vi "GetINIPathForAModule.vi"(8 "error in (no error)":errorcluster, 10 "Module":string, 11 "Test":refnum<class "Test.lvclass">) -> (0 "Error out":errorcluster, 2 "INI File":path, 3 "Test Class out":refnum<class "Test.lvclass">)   [LabVIEW 2018, in "Test.lvclass"]
uses:
  Test.lvclass
  Test.lvclass/Test.ctl
  Accessors/Read ErrorSeverity.vi
  Accessors/Read PluginPathArray.vi
  Accessors/Read PluginIndex.vi
  Accessors/Read ModuleList.vi
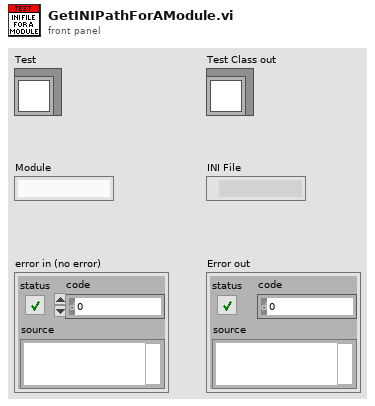
[diagram p1: front panel]
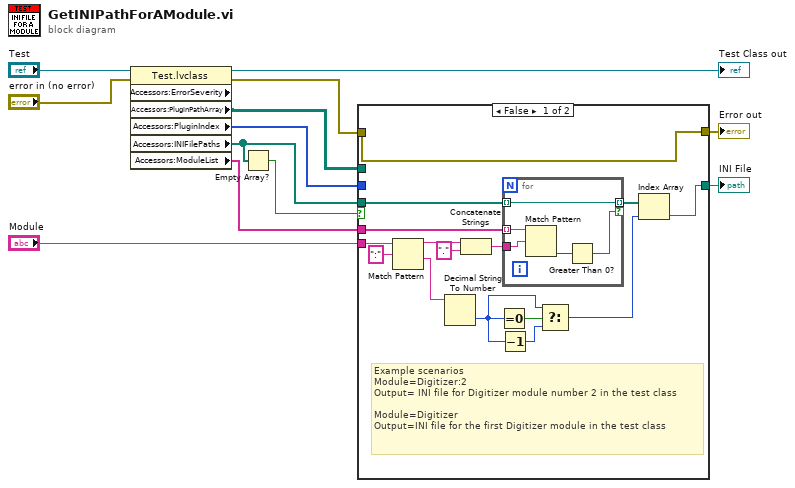
[diagram p0: block diagram]
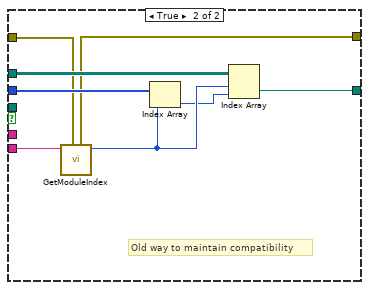
[diagram p2: hidden frame]
diagram:
  n1 = property class="Test.lvclass" props=["Accessors:ErrorSeverity", "Accessors:PluginPathArray", "Accessors:PluginIndex", "Accessors:INIFilePaths", "Accessors:ModuleList"](reference="Test", error in="error in (no error)") -> (reference out=→"Test Class out":refnum<class "Test.lvclass">, error out=w9:errorcluster, "Accessors:PluginPathArray"=w8:path[][], "Accessors:PluginIndex"=w7:u32[], "Accessors:INIFilePaths"=w6:path[], "Accessors:ModuleList"=w4:string[])  [unwired: 1 out]
  n2 = Empty Array?(array=w6) -> (empty?=w5:bool)
  n3 = case shown="False" w5 {
    tunnel: w7 -> [_ w40]
    tunnel: w8 -> [_ w39]
    tunnel: [w18 w38] -> w2
    tunnel: "Module" -> [w27 w37]
    tunnel: [w17 w36] -> w1
    tunnel: w9 -> [w17 w33]
    tunnel: w6 -> [w21 _]
    tunnel: w4 -> [w23 _]
    frame False {
      # "Example scenarios\nModule=Digitizer:2\nOutput= INI file for Digitizer module number 2 in the test class\n\nModule=Digitizer\nOutput=INI file for the first Digitizer module in the test class"
      n4 = Match Pattern(string=w27, regular expression=":") -> (before substring=w25:string, after substring=w20:string)  [unwired: 1 in, 2 out]
      n5 = Decimal String To Number(string=w20) -> (number=w15:i32)  [unwired: 2 in, 1 out]
      n6 = Concatenate Strings(w25, "." ("string")) -> (w22:string)
      n7 = Equal To 0?(x=w15) -> (x = 0?=w16:bool)
      n8 = Decrement(x=w15) -> (x-1=w14:i32)
      n9 = for {
        tunnel: w23 -> [w32] mode=indexing
        tunnel: w22 -> [w31]
        tunnel: w21 -> [w29] mode=indexing
        tunnel: [w29] -> w19 mode=indexing if=w28
        n10 = Match Pattern(string=w32, regular expression=w31) -> (offset past match=w30:i32)  [unwired: 1 in, 3 out]
        n11 = Greater Than 0?(x=w30) -> (x > 0?=w28:bool)
      }
      n12 = Select(t=w15, s=w16, f=w14) -> (s? t:f=w13:i32)
      n13 = Index Array(array=w19, index=w13) -> (element=w18:path)
    }
    frame True {
      # "Old way to maintain compatibility"
      n14 = call "GetModuleIndex.vi"("Error In"=w33, "ModuleType"=w37) -> ("ModuleIndex"=w35:i32, "Error"=w36:errorcluster)  [unwired: 8 in]
      n15 = Index Array(array=w40, index=w35) -> (element=w34:u32)
      n16 = Index Array(array=w39, index (row)=w35, index (col)=w34) -> (element=w38:path)
    }
  }
  "INI File" <- w2
  "Error out" <- w1
